vi "Move stage to diode position.vi"() -> (0 "error out":errorcluster)   [LabVIEW 2011]
uses:
  <vilib>/Utility/file.llb/Read From Spreadsheet File (string).vi
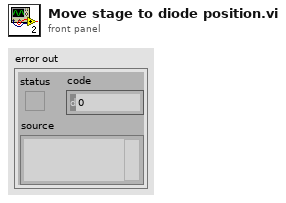
[diagram p1: front panel]
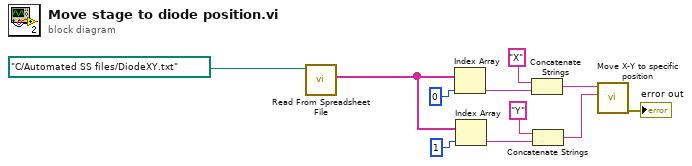
[diagram p0: block diagram]
diagram:
  n1 = call-poly <vilib>:"Read From Spreadsheet File.vi"("file path (dialog if empty)"=path "C:/Automated SS files/DiodeXY.txt") -> ("first row"=w4:string[])  [unwired: 6 in, 4 out]
  n2 = Index Array(array=w4, index=0) -> (element=w5:string)
  n3 = Index Array(array=w4, index=1) -> (element=w6:string)
  n4 = Concatenate Strings("X", w5) -> (w9:string)
  n5 = Concatenate Strings("Y", w6) -> (w10:string)
  n6 = call "Move X-Y to specific position.vi"("position 2"=w10, "position 1"=w9) -> ("error out 3"=→"error out":errorcluster)  [unwired: 5 in, 4 out]
